vi "ClientGlobals.vi"() -> ()   [LabVIEW 2017, in "Client.lvlib"]
uses:
  Client.lvlib
panel:
  in  "INI Path":path
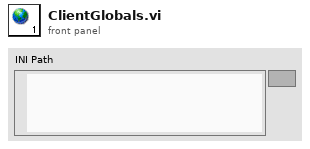
[diagram p1: front panel]
diagram:
